vi "rot - Givens Rotation.vi"   [LabVIEW 2017, in "NI_AALBLAS.lvlib"]
doc: "Applies a Givens rotation to a set of points."
uses:
  <vilib>/Analysis/NI_AALBLAS.lvlib
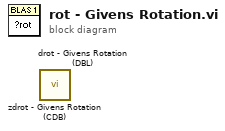
[diagram p0: block diagram]
diagram:
  n1 = call <vilib>:"zdrot - Givens Rotation (CDB).vi"() -> ()  [unwired: 9 in, 3 out]
  n2 = call <vilib>:"drot - Givens Rotation (DBL).vi"() -> ()  [unwired: 9 in, 3 out]
